vi "Estimate_State-Space_Model_from_FRFs_Parameter_Adjustment_v2.vi"() -> ()   [LabVIEW 2022 SP3]
doc: "This example demonstrates how to use frequency-domain data to estimate a state-space model. \n\n<B>Instructions:</B>\n1) Run this VI.\n2) Observe how the simulated frequency response matches the measured frequency response.\n3) Change the orders of the models, and observe how these changes affect the estimation error."
uses:
  <vilib>/addons/System Identification/Model Typedefs.llb/SI Pole-Zero Plot.ctl
  <vilib>/addons/System Identification/Frequency Domain Estimation.llb/SI Estimate Discrete State-Space Model from FRF (SISO Arbitrary).vi
  <vilib>/addons/System Identification/NI_SysID.lvlib
panel:
  in  "confidence level (%)":dbl=99.0 format="%_2f"
  out "pole-zero plot":T1
  in  "name or relative path":path=path "C:/Users/LAV-UFSC/OneDrive - UFSC/Documents/LAV - TCC/Dados-Experimentos/25-04/frf_2.txt"
  in  "noise subspace (%)":dbl=78.0
  in  "FRF format":T2={"dB on? (F)"=FALSE, "unwrap phase? (F)"=FALSE, "convert to degree? (F)"=TRUE}
  out "Phase Response":cluster{"frequency":dbl[], "amplitude":dbl[]}[](graph)
  out "Magnitude Response":cluster{"frequency":dbl[], "amplitude":dbl[]}[](graph)
  in  "Order":i32=9
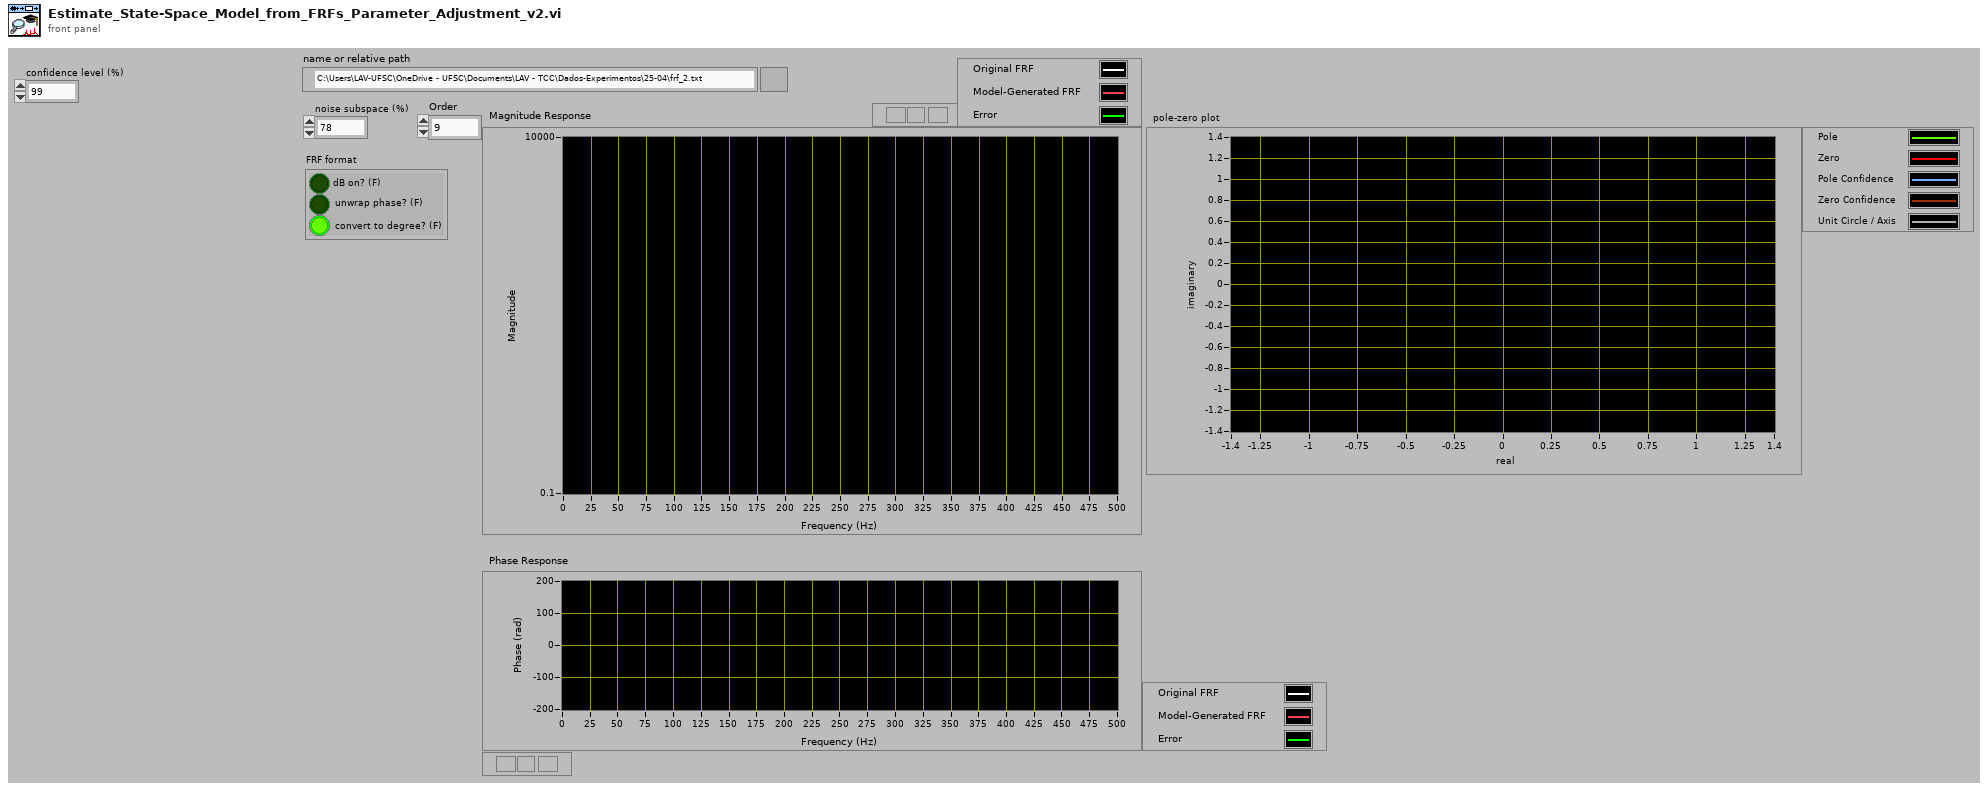
[diagram p1: front panel]
types:
  T1 = typedef "NI_SysID.lvlib/SI Pole-Zero Plot.ctl" = cluster{"frequency":dbl[], "amplitude":dbl[]}[]
  T2 = cluster{"dB on? (F)":bool, "unwrap phase? (F)":bool, "convert to degree? (F)":bool}
  T3 = cluster{"start frequency":dbl, "end frequency":dbl, "num of freq bins":i32, "interval type":u16}
  T4 = typedef "NI_SysID.lvlib/si_generic model.ctl" = cluster{"attributes":cluster{"version":string, "model type":T5, "input names":string[], "output names":string[], "notes":string}, "coefficients":cluster{"A ":dbl[][][], "B":dbl[][][], "F":dbl[][][], "C":dbl[][][], "D":dbl[][][]}, "std deviations":cluster{"A ":dbl[][][], "B":dbl[][][], "F":dbl[][][], "C":dbl[][][], "D":dbl[][][]}, "coefficients covariance":dbl[][][], "noise variance":dbl[][], "fs":dbl, "system info":cluster{"number of inputs":i32, "number of outputs":i32, "A order":i32[][], "B order":i32[][], "F order":i32[][], "C order":i32[][], "D order":i32[][], "Delays":i32[][]}, "kalman gain":dbl[][], "initial state":dbl[], "trans func":cluster{"betas":dbl[], "alphas":dbl[]}[][], "zeros-poles":cluster{"zeros":cdb[], "poles":cdb[], "gain":dbl}[][], "std of trans func":cluster{"betas":dbl[], "alphas":dbl[]}[][], "std of zeros-poles":cluster{"zeros":cdb[], "poles":cdb[], "gain":dbl}[][], "trans func (noise)":cluster{"betas":dbl[], "alphas":dbl[]}[][], "std of trans func (noise)":cluster{"betas":dbl[], "alphas":dbl[]}[][], "zeros-poles (noise)":cluster{"zeros":cdb[], "poles":cdb[], "gain":dbl}[][], "std of zeros-poles (noise)":cluster{"zeros":cdb[], "poles":cdb[], "gain":dbl}[][], "Symbolic State Space Model":cluster{"Symbolic A":string[][], "Symbolic B":string[][], "Symbolic C":string[][], "Symbolic D":string[][], "Symbolic K":string[][], "Symbolic Initial State":string[]}, "delay":dbl[][], "variables":T6, "grey trans func spec":cluster{"orders of TF model":cluster{" num order":i32, "den order":i32}, "# of zeros/poles at origin":cluster{"zeros/poles":u16, "number ":i32}, "delay initial?":bool, "gain initial?":bool}}
  T5 = typedef "NI_SysID.lvlib/SI Model Type.ctl" = u16
  T6 = typedef "NI_SysID.lvlib/si_variables.ctl" = cluster{"name":string, "initial guess":dbl, "upper limit":dbl, "lower limit":dbl, "value":dbl}[]
  T7 = typedef "NI_SysID.lvlib/si_Bode Phase Plot.ctl" = cluster{"frequency":dbl[], "amplitude":dbl[]}[]
  T8 = typedef "NI_SysID.lvlib/si_Bode Magnitude Plot.ctl" = cluster{"frequency":dbl[], "amplitude":dbl[]}[]
  T9 = cluster{"frequency":dbl[], "phase (wrapped)":dbl[]}
  T10 = cluster{"frequency":dbl[], "phase (wrapped)":dbl[]}[]
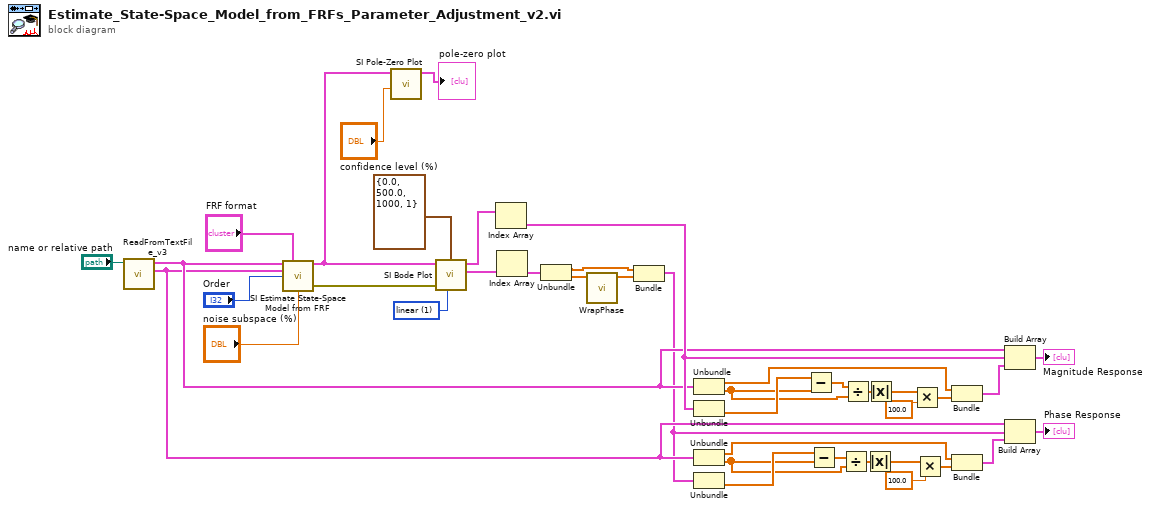
[diagram p0: block diagram]
diagram:
  w32 = u16 1 items=["dB", "linear"] ("magnitude unit")
  n1 = call "ReadFromTextFile_v3.vi"("name or relative path"="name or relative path") -> ("Phase"=w14:cluster{dbl[], dbl[]}, "Magnitude"=w15:cluster{dbl[], dbl[]})  [unwired: 6 in, 2 out]
  n2 = call-poly <vilib>:"SI Estimate State-Space Model from FRF.vi"("FRF magnitude"=w15, "FRF format"="FRF format", "FRF phase"=w14, "number of states"="Order", "noise subspace (%)"="noise subspace (%)") -> ("system model out"=w31:T4, "error out"=w33:errorcluster)  [unwired: 3 in, 6 out]
  n3 = call <vilib>:"SI Pole-Zero Plot.vi"("confidence level (%)"="confidence level (%)", "system model"=w31) -> ("pole-zero plot"=→"pole-zero plot":T1)  [unwired: 8 in, 1 out]
  n4 = call <vilib>:"SI Bode Plot.vi"("magnitude unit"=w32, "freq info"=T3 {"start frequency"=0.0, "end frequency"=500.0, "num of freq bins"=1000, "interval type"=1}, "error in (no error)"=w33, "system model"=w31) -> ("Bode phase plot"=w27:T7, "Bode magnitude plot"=w28:T8)  [unwired: 3 in, 3 out]
  n5 = Index Array(array=w28) -> (element=w16:cluster{"frequency":dbl[], "amplitude":dbl[]})  [unwired: 1 in]
  n6 = Index Array(array=w27) -> (element=w5:cluster{"frequency":dbl[], "amplitude":dbl[]})  [unwired: 1 in]
  n7 = Unbundle(w5) -> ("frequency"=w1:dbl[], "amplitude"=w3:dbl[])
  n8 = call "WrapPhase.vi"("phase (upwrapped)"=w3) -> ("phase (wrapped)"=w2:dbl[])  [unwired: 10 in]
  n9 = Bundle("frequency"=w1, "phase (wrapped)"=w2) -> (w4:T9)  [unwired: 1 in]
  n10 = Unbundle(w15) -> (w24:dbl[], w25:dbl[])
  n11 = Unbundle(w16) -> ("amplitude"=w26:dbl[])  [unwired: 1 out]
  n12 = Unbundle(w14) -> (w6:dbl[], w17:dbl[])
  n13 = Unbundle(w4) -> ("phase (wrapped)"=w22:dbl[])  [unwired: 1 out]
  n14 = Subtract(x=w26, y=w25) -> (x-y=w20:dbl[])
  n15 = Subtract(x=w22, y=w17) -> (x-y=w18:dbl[])
  n16 = Divide(x=w18, y=w17) -> (x/y=w19:dbl[])
  n17 = Divide(x=w20, y=w25) -> (x/y=w23:dbl[])
  n18 = Absolute Value(x=w19) -> (abs(x)=w7:dbl[])
  n19 = Absolute Value(x=w23) -> (abs(x)=w9:dbl[])
  n20 = Multiply(x=w9, y=100.0) -> (x*y=w12:dbl[])
  n21 = Multiply(x=w7, y=100.0) -> (x*y=w11:dbl[])
  n22 = Bundle(w24, w12) -> (w21:cluster{dbl[], dbl[]})  [unwired: 1 in]
  n23 = Bundle(w6, w11) -> (w13:cluster{dbl[], dbl[]})  [unwired: 1 in]
  n24 = Build Array(w15, w16, w21) -> (→"Magnitude Response":cluster{"frequency":dbl[], "amplitude":dbl[]}[])
  n25 = Build Array(w14, w4, w13) -> (→"Phase Response":T10)
